vi "Datalogging.vi"(0 "Logging Data":T1, 1 "Log File Reference":refnum<file>, 2 "Match Ended?":bool, 3 "Second Passed?":bool) -> (8 "File Closed?":bool)   [LabVIEW 2015]
uses:
  <vilib>/Utility/file.llb/Write Delimited Spreadsheet (DBL).vi
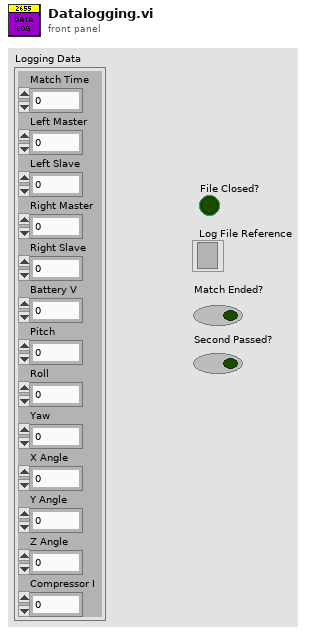
[diagram p1: front panel]
types:
  T1 = cluster{"Match Time":dbl, "Left Master":dbl, "Left Slave":dbl, "Right Master":dbl, "Right Slave":dbl, "Battery V":dbl, "Pitch":dbl, "Roll":dbl, "Yaw":dbl, "X Angle":dbl, "Y Angle":dbl, "Z Angle":dbl, "Compressor I":dbl}
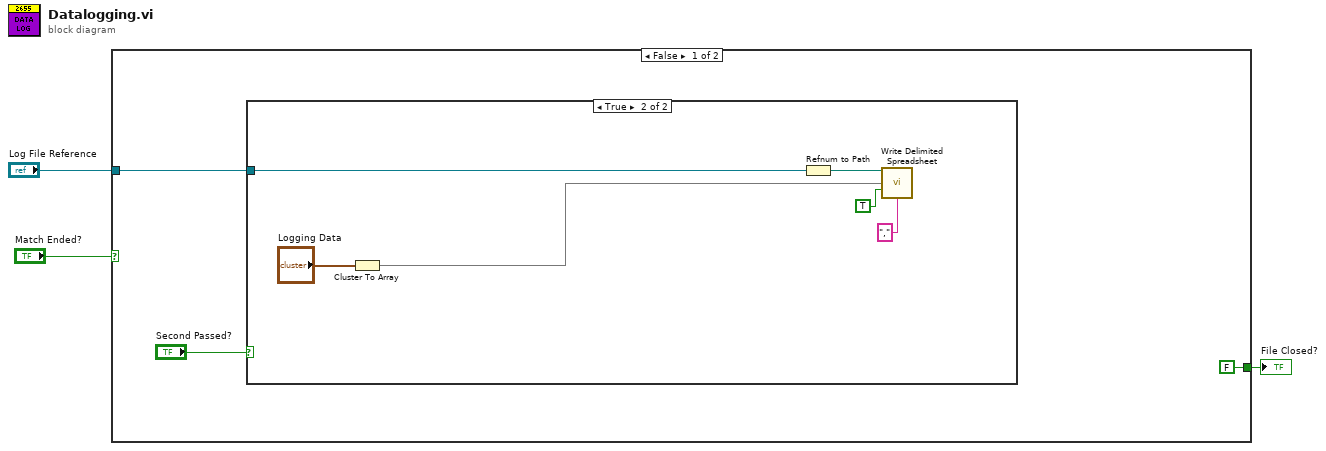
[diagram p0: block diagram]
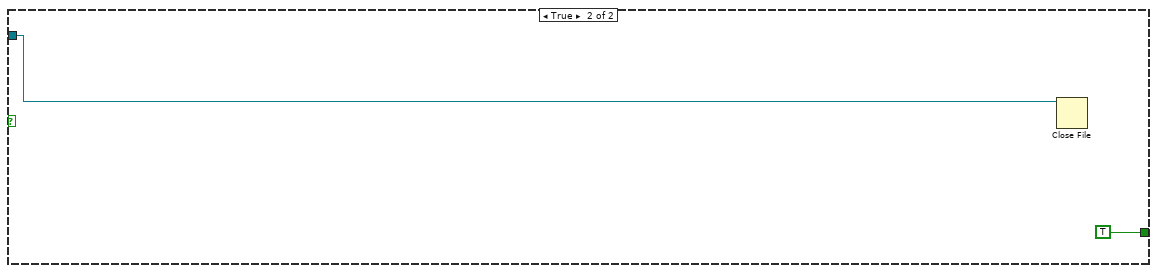
[diagram p3: hidden frame]
diagram:
  n1 = case shown="False" "Match Ended?" {
    tunnel: "Log File Reference" -> [w5 w14]
    tunnel: [FALSE TRUE] -> w1
    frame False {
      n2 = case shown="True" "Second Passed?" {
        tunnel: w5 -> [_ w10]
        frame False {
        }
        frame True {
          n3 = Cluster To Array(cluster="Logging Data") -> (array=w8:dbl[])
          n4 = Refnum to Path(1:w10) -> (0:w9:path)
          n5 = call-poly <vilib>:"Write Delimited Spreadsheet.vi"("file path (dialog if empty)"=w9, "1D data"=w8, "append to file? (F)"=TRUE, "delimiter (\\t)"="," ("delimiter (\\t)")) -> ()  [unwired: 10 in, 2 out]
        }
      }
    }
    frame True {
      n6 = Close File(refnum=w14) -> ()  [unwired: 1 in, 2 out]
    }
  }
  "File Closed?" <- w1
